vi "Untitled 1.vi"() -> ()   [LabVIEW 2014]
uses:
  <vilib>/Aledyne-TSXperts/Arduino Compatible Compiler for LabVIEW/Arduino Compatible Compiler for LabVIEW.lvlib
panel:
  in  "Speed":u32=9600
  out "error out":errorcluster
  in  "error in (no error)":errorcluster
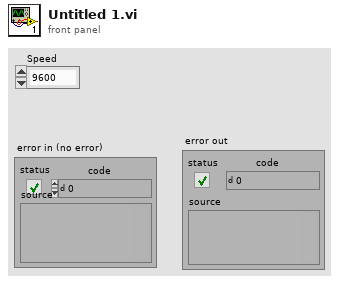
[diagram p1: front panel]
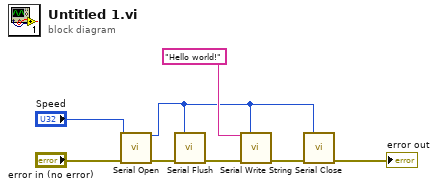
[diagram p0: block diagram]
diagram:
  n1 = call <vilib>:"Serial Open.vi"("Speed"="Speed", "error in (no error)"="error in (no error)") -> ("Instance"=w2:u8, "error out"=w8:errorcluster)  [unwired: 12 in]
  n2 = call <vilib>:"Serial Flush.vi"("Instance"=w2, "error in (no error)"=w8) -> ("error out"=w7:errorcluster)  [unwired: 13 in]
  n3 = call <vilib>:"Serial Write String.vi"("String"="Hello world!", "Instance"=w2, "error in (no error)"=w7) -> ("error out"=w6:errorcluster)  [unwired: 12 in]
  n4 = call <vilib>:"Serial Close.vi"("Instance"=w2, "error in (no error)"=w6) -> ("error out"=→"error out":errorcluster)  [unwired: 13 in]
